vi "Start Sequence.vi"(8 "error in (no error)":errorcluster, 11 "Sequencer in":refnum<class "Sequencer.lvclass">) -> (0 "error out":errorcluster, 3 "Sequencer out":refnum<class "Sequencer.lvclass">)   [LabVIEW 2024, in "Ramses Sequencer.lvlib" / "Sequencer.lvclass"]
uses:
  Sequencer.lvclass
  typedef/Sequencer State -- enum.ctl
  Program Files (x86)/Enterative/Ramses Framework/Ramses Framework.lvlibp/Service/Service.lvclass
  C:/Program Files (x86)/Enterative/Ramses Framework/Ramses Framework.lvlibp/Service/Service.lvclass
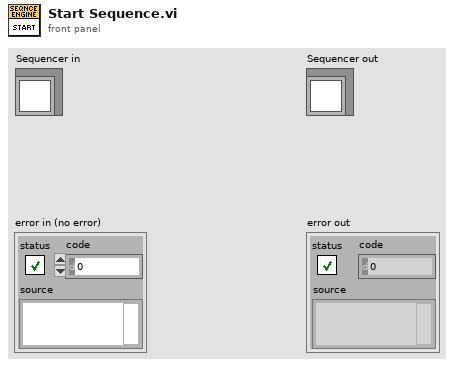
[diagram p1: front panel]
types:
  T1 = typedef "Ramses Sequencer.lvlib/Sequencer.lvclass/Sequencer State -- enum.ctl" = enum16{"Idle", "Running", "Paused", "Complete"}
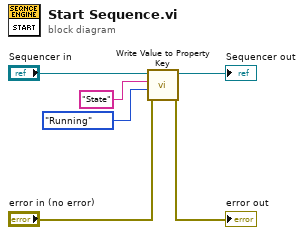
[diagram p0: block diagram]
diagram:
  n1 = call "Write Value to Property Key.vi"("error in (no error)"="error in (no error)", "Value"=Sequencer_State_--_enum."Running" ("Sequencer State"), "Key"="State", "Service in"="Sequencer in") -> ("error out"=→"error out":errorcluster, "Service out"=→"Sequencer out":refnum<class "Sequencer.lvclass">)  [unwired: 6 in]
